vi "CELSIUS TO FARHENHEIT.vi"() -> ()   [LabVIEW 2019]
panel:
  out "TEMPERATURE IN FARHENHEIT":dbl(slide) scale=0.0..500.0
  in  "TEMPERATURE IN CELSIUS":dbl(slide)=100.26109660574414 scale=0.0..200.0
  # "CONVERSION OF CELSIUS TO FARHENHEIT"
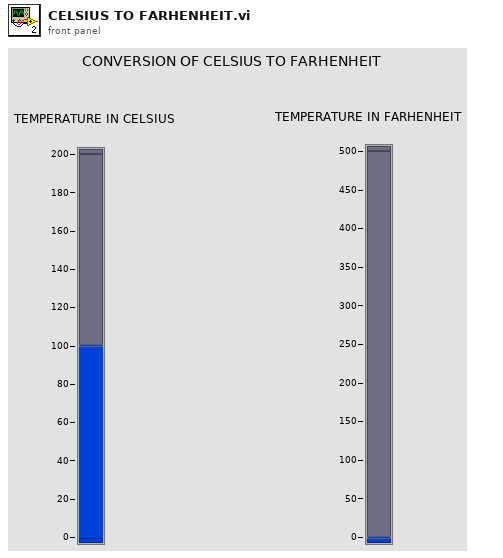
[diagram p1: front panel]
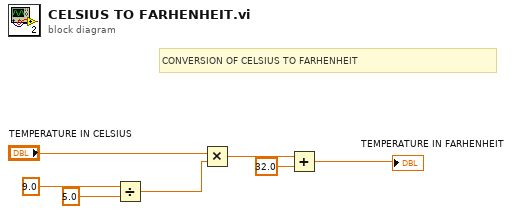
[diagram p0: block diagram]
diagram:
  # "CONVERSION OF CELSIUS TO FARHENHEIT"
  n1 = Divide(x=9.0, y=5.0) -> (x/y=w7:dbl)
  n2 = Multiply(x="TEMPERATURE IN CELSIUS", y=w7) -> (x*y=w4:dbl)
  n3 = Add(x=w4, y=32.0) -> (x+y=→"TEMPERATURE IN FARHENHEIT":dbl)
